vi "headers.build.vi"(9 "request specific headers":T1[](array[typedef]), 10 "default headers":T1[](array[typedef])) -> (2 "Headers JSON":string)   [LabVIEW 2020, in "reqwest.lvclass"]
uses:
  reqwest.lvclass
  header.ctl
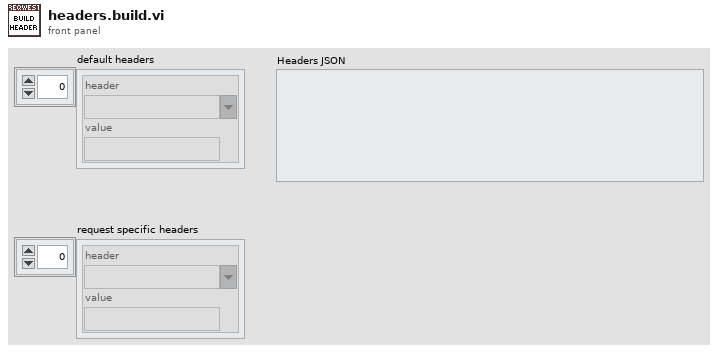
[diagram p1: front panel]
types:
  T1 = typedef "reqwest.lvclass/header.ctl" = cluster{"header":string, "value":string}
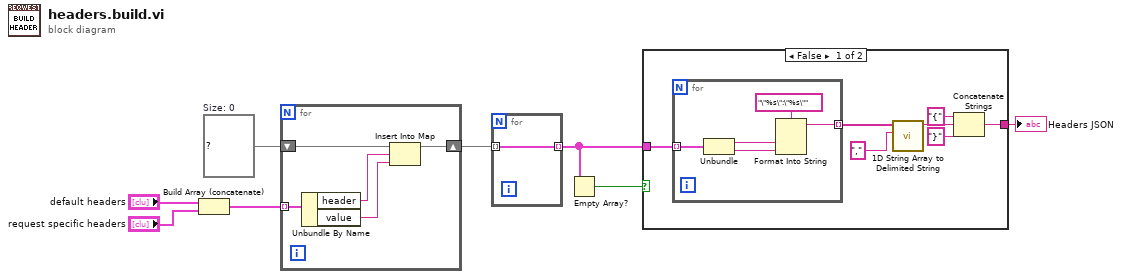
[diagram p0: block diagram]
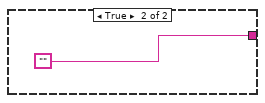
[diagram p2: hidden frame]
diagram:
  w6 = map{string, string} {}  # Size: 0
  n1 = Build Array (concatenate)("default headers", "request specific headers") -> (w5:T1[])
  n2 = for {
    shift-right: [w12] -> w4
    shift-left: w6 -> [w13]
    tunnel: w5 -> [w11] mode=indexing
    n3 = Unbundle By Name(w11) -> ("header"=w10:string, "value"=w9:string)
    n4 = Insert Into Map(map in=w13, key=w10, value=w9) -> (map out=w12:map{string, string})  [unwired: 2 out]
  }
  n5 = for {
    tunnel: w4 -> [w14] mode=indexing
    tunnel: [w14] -> w3 mode=indexing
  }
  n6 = Empty Array?(array=w3) -> (empty?=w7:bool)
  n7 = case shown="False" w7 {
    tunnel: [w15 ""] -> w8
    tunnel: w3 -> [w21 _]
    frame False {
      n8 = for {
        tunnel: w21 -> [w26] mode=indexing
        tunnel: [w22] -> w20 mode=indexing
        n9 = Unbundle(w26) -> (w24:string, w23:string)
        n10 = Format Into String(format string="\"%s\":\"%s\"", w24, w23) -> (resulting string=w22:string)  [unwired: 2 in, 1 out]
      }
      n11 = call <vilib>:"1D String Array to Delimited String.vi"("delimiter"=",", "string array"=w20) -> ("delimited string"=w18:string)  [unwired: 9 in]
      n12 = Concatenate Strings("{" ("string"), w18, "}" ("string")) -> (w15:string)
    }
    frame True {
    }
  }
  "Headers JSON" <- w8
